vi "ReceiveWithData.vi"(8 "error in (no error)":errorcluster, 11 "Receiver in":refnum<class "Receiver.lvclass">) -> (0 "error out":errorcluster, 1 "Message Status":bool, 2 "Variant Data":variant, 3 "Receiver out":refnum<class "Receiver.lvclass">)   [LabVIEW 2023, in "Receiver.lvclass"]
uses:
  Receiver.lvclass
  Receiver.lvclass/Receiver.ctl
  Data/Data.lvclass
  Communication/Communication.lvclass
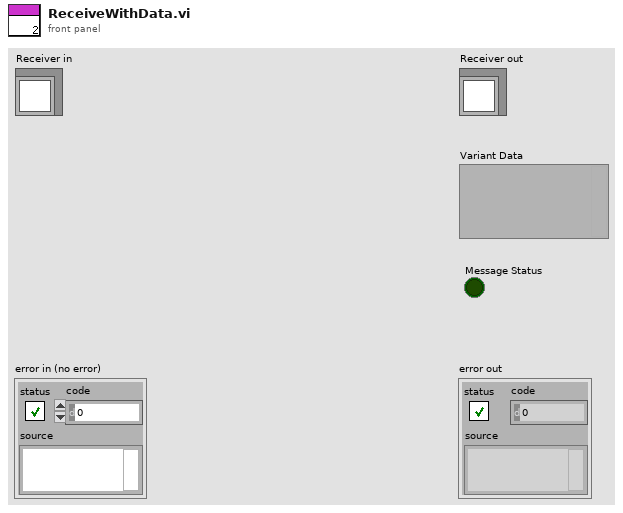
[diagram p1: front panel]
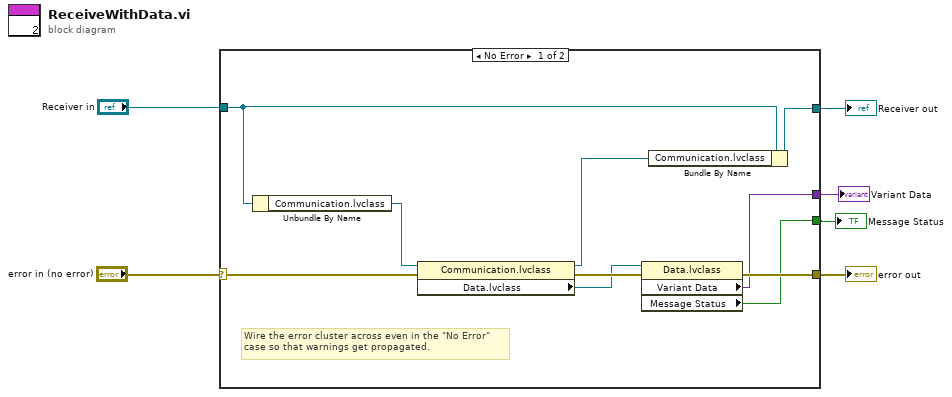
[diagram p0: block diagram]
diagram:
  n1 = case shown="No Error" "error in (no error)" {
    selector: "error in (no error)" -> [w14 w18]
    tunnel: [w11 w18] -> w5
    tunnel: [w15 w17] -> w3
    tunnel: "Receiver in" -> [w13 w17]
    tunnel: [w8 _] -> w2
    tunnel: [w7 _] -> w1
    frame No Error {
      # "Wire the error cluster across even in the \"No Error\"\ncase so that warnings get propagated."
      n2 = Unbundle By Name(w13) -> ("Communication.lvclass"=w12:refnum<class "Communication.lvclass">)
      n3 = property class="Communication.lvclass"(reference=w12, error in=w14) -> (reference out=w9:refnum<class "Communication.lvclass">, error out=w16:errorcluster, "Data.lvclass"=w10:refnum<class "Data.lvclass">)
      n4 = property class="Data.lvclass"(reference=w10, error in=w16) -> (error out=w11:errorcluster, "Variant Data"=w8:variant, "Message Status"=w7:bool)  [unwired: 1 out]
      n5 = Bundle By Name(cluster=w13, "Communication.lvclass"=w9) -> (w15:refnum<class "Receiver.lvclass">)
    }
    frame Error {
    }
  }
  "error out" <- w5
  "Receiver out" <- w3
  "Variant Data" <- w2
  "Message Status" <- w1
